vi "Bodies_GetVecInXYZ0.vi"(8 "error in (no error)":errorcluster, 9 "Body ID":i32, 10 "Vector":dbl[](array[numeric]), 11 "Bodies.lvclass":refnum<class "Bodies.lvclass">) -> (0 "error out":errorcluster, 2 "Vector in GCS":dbl[](array[numeric]) format="%#.6f", 3 "Bodies.lvclass 2":refnum<class "Bodies.lvclass">)   [LabVIEW 2015, in "Bodies.lvclass"]
uses:
  Bodies.lvclass
  Bodies.lvclass/Bodies.ctl
  <vilib>/Analysis/Matrix/Numeric/Conversions/Array To Matrix - RA2.vi
  <vilib>/Analysis/BLAS.llb/dgemv - General Matrix-Vector Product (DBL).vi
  <vilib>/Analysis/NI_AALBLAS.lvlib
  <vilib>/Analysis/NI_AALBase.lvlib
  <vilib>/Analysis/Matrix/NI_Matrix.lvlib
  <vilib>/Analysis/baseanly.llb/A x Vector.vi
panel:
  # "Convert vectors like a force or moment"
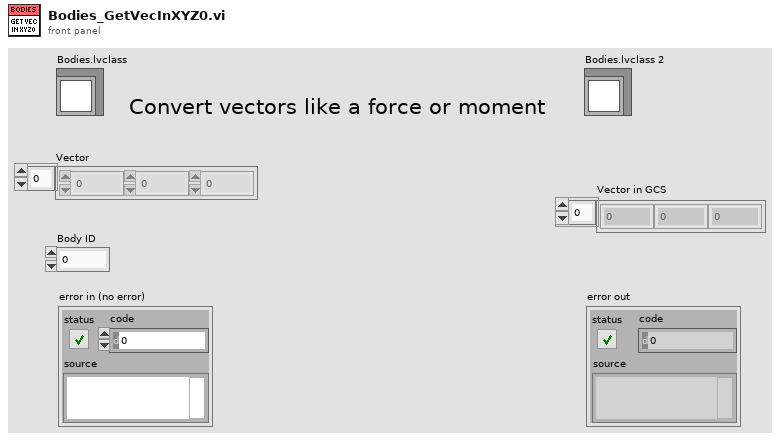
[diagram p1: front panel]
types:
  T1 = typedef "NI_Matrix.lvlib/RealMatrix.ctl" = dbl[][]
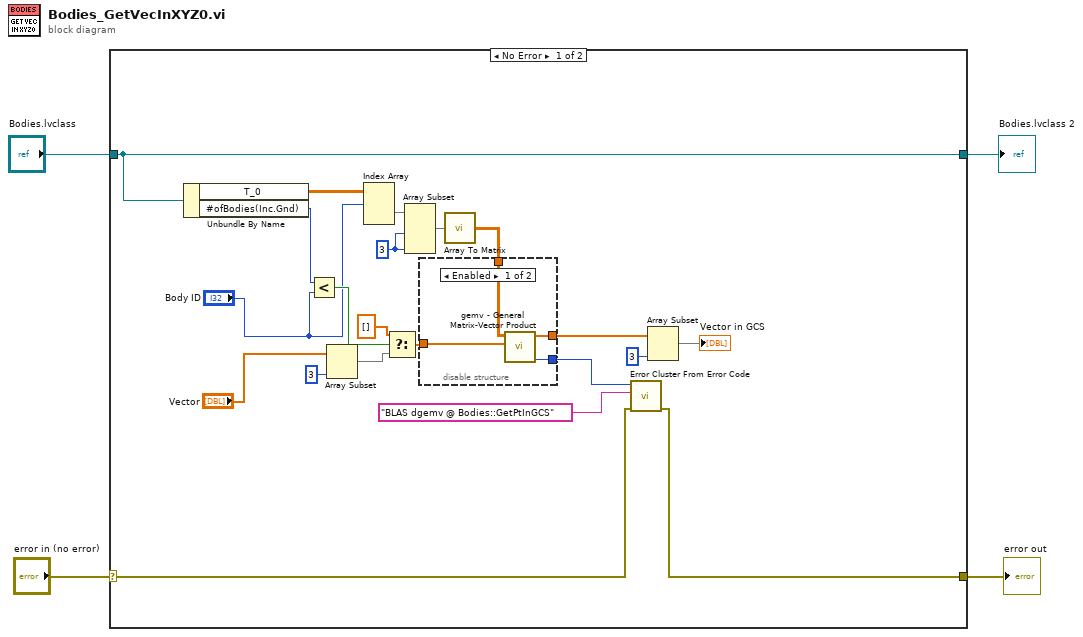
[diagram p0: block diagram]
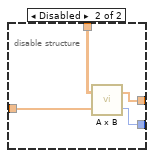
[diagram p2: hidden frame]
diagram:
  n1 = case shown="No Error" "error in (no error)" {
    selector: "error in (no error)" -> [w19 w35]
    tunnel: "Bodies.lvclass" -> [w18 w34]
    tunnel: [w25 w35] -> w3
    tunnel: [w18 w34] -> w1
    frame No Error {
      w7 = 3 ("length")
      n2 = Unbundle By Name(w18) -> ("T_0"=w17:dbl[][][], "#ofBodies(Inc.Gnd)"=w15:i32)
      n3 = Less?(x=w15, y="Body ID") -> (x < y?=w14:bool)
      n4 = Array Subset(array="Vector", length=3) -> (w10:dbl[])  [unwired: 1 in]
      n5 = Index Array(array=w17, index (dim 0)="Body ID") -> (element=w9:dbl[][])  [unwired: 2 in]
      n6 = Select(t=dbl[] [], s=w14, f=w10) -> (s? t:f=w13:dbl[])
      n7 = Array Subset(array=w9, length (row)=w7, length (col)=w7) -> (w8:dbl[][])  [unwired: 2 in]
      n8 = call-poly <vilib>:"Array To Matrix.vi"("Real 2D Array"=w8) -> ("Real Matrix"=w16:T1)
      n9 = disable-structure shown="Enabled" {
        disable-tunnel: [w29 w30] -> w23
        disable-tunnel: [w28 w31] -> w22
        disable-tunnel: w16 -> [w27 w33]
        disable-tunnel: w13 -> [w26 w32]
        frame Enabled {
          n10 = call-poly <vilib>:"gemv - General Matrix-Vector Product.vi"("x"=w26, "A"=w27) -> ("error"=w29:i32, "dgemv"=w28:dbl[])  [unwired: 8 in]
        }
        frame Disabled {
          n11 = call-poly <vilib>:"A x B.vi"("Vector"=w32, "A"=w33) -> ("error"=w30:i32, "A x Vector"=w31:dbl[])
        }
      }
      n12 = call <vilib>:"Error Cluster From Error Code.vi"("error in (no error)"=w19, "error message (\"\")"="BLAS dgemv @ Bodies::GetPtInGCS" ("error source (\" \")"), "error code (0)"=w23) -> ("error out"=w25:errorcluster)  [unwired: 6 in]
      n13 = Array Subset(array=w22, length=3) -> (→"Vector in GCS":dbl[])  [unwired: 1 in]
    }
    frame Error {
    }
  }
  "error out" <- w3
  "Bodies.lvclass 2" <- w1
